vi "FindPeak.vi"(11 "Input XY":T1) -> (1 "Peak Count":dbl, 2 "output Line":T1, 3 "Peak Position":dbl)   [LabVIEW 2020]
uses:
  <vilib>/Analysis/3filter.llb/Butterworth Filter (DBL).vi
  <vilib>/Analysis/NI_AALBase.lvlib
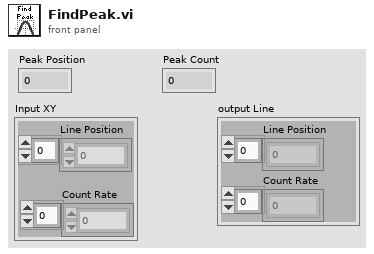
[diagram p1: front panel]
types:
  T1 = cluster{"Line Position":dbl[], "Count Rate":dbl[]}
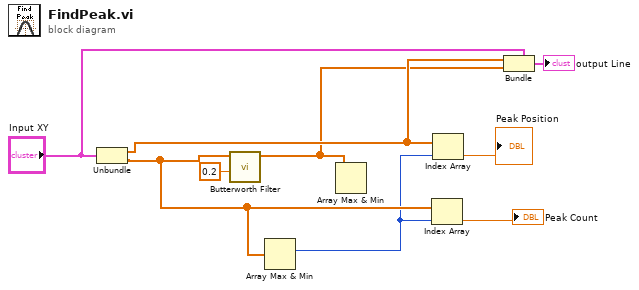
[diagram p0: block diagram]
diagram:
  n1 = Unbundle("Input XY") -> ("Line Position"=w7:dbl[], "Count Rate"=w2:dbl[])
  n2 = call-poly <vilib>:"Butterworth Filter.vi"("high cutoff freq: fh"=0.2, "X"=w2) -> ("Filtered X"=w6:dbl[])  [unwired: 6 in, 1 out]
  n3 = Array Max & Min(array=w2) -> (max index (indices)=w1:i32)  [unwired: 3 out]
  n4 = Array Max & Min(array=w6) -> ()  [unwired: 4 out]
  n5 = Index Array(array=w2, index=w1) -> (element=→"Peak Count":dbl)
  n6 = Index Array(array=w7, index=w1) -> (element=→"Peak Position":dbl)
  n7 = Bundle(cluster="Input XY", "Line Position"=w7, "Count Rate"=w6) -> (→"output Line":T1)
